vi "SerialCommand.vi"(4 "Received":refnum<k21>, 5 "ReceivedBuffer":refnum<k21>, 6 "Transmitted":refnum<k21>, 7 "Out":refnum<k21>, 8 "error in (no error)":errorcluster, 9 "CommandFIFO":refnum<k21>, 10 "Command":u8, 11 "Port":refnum<k21>) -> (0 "error out":errorcluster)   [LabVIEW 2023]
uses:
  <vilib>/rvi/DataTransferAndStorage/Container/Common/niFpgaContainerExecOnDevCompGetState.vi
  <vilib>/rvi/Emulation/niFpgaEmulationIsFPGAContextNoSignature.vi
  <vilib>/rvi/Emulation/niFpgaSctlEmulationGetInTimedLoop.vi
  <vilib>/rvi/errors/niFpgaSetErrorForExecOnDevCompSimple.vi
  <vilib>/rvi/eio/common/nirviEmuReportErrorAndStop.vi
  <vilib>/rvi/DataTransferAndStorage/Container/Common/niFpgaContainerGetUniqueNameForEmu.vi
  <vilib>/rvi/FIFO/Fifo_Resource/nirvififoEmulationSetSize.vi
  <vilib>/rvi/FIFO/Fifo_Resource/nirviFifoEmulationQueueMgr.vi
  <instcachedir>/0/nirviFifoEmulationQueueMgr_E5CAEC123FF24DC58D834DCA3CDAA9B5.lvgen/nirviFifoEmulationQueueMgr_E5CAEC123FF24DC58D834DCA3CDAA9B5_002.vi
  <vilib>/rvi/FIFO/Fifo_Resource/nirvififoEmulationDetermineInputValidOut.vi
  <vilib>/rvi/FIFO/Fifo_Resource/nirvififoEmulationCreateLock.vi
  <vilib>/rvi/Emulation/niFpgaProcessEmulError.vi
  <vilib>/rvi/FIFO/Fifo_Resource/nirvififoEmulationObtainLock.vi
  <vilib>/rvi/FIFO/Fifo_Resource/nirvififoEmulationReleaseLock.vi
  <vilib>/rvi/occurrence/nirviWaitOnOccurrenceBase.vi
  <vilib>/rvi/errors/nirviReportUnexpectedCaseInternalError.vi
  <vilib>/rvi/errors/nirviReportUnexpectedCaseInternalError (U32).vi
  <vilib>/Utility/error.llb/Clear Errors.vi
  <vilib>/eio/utilities/niEioResolveVilibRelativePath.vi
  <vilib>/rvi/interface/RandomDataEmulation/niFpgaRandomDataHandleErrors.vi
  <vilib>/rvi/Memory/Memory_Emulation/niFpgaMemoryEmulationCacheClearOnFirstRun.vi
  <vilib>/rvi/Memory/Memory_Emulation/nirvimemoryEmulationManagerCache_MakeExclusive.vi
  <vilib>/rvi/Memory/Memory_Emulation/niFpgaMemoryEmulationValidateCache.vi
  <vilib>/rvi/Memory/Memory_Emulation/nirvimemoryEmulationManagerCache_InsertValue.vi
  <vilib>/rvi/Memory/Memory_Emulation/nirvimemoryEmulationManagerCache_ReleaseExclusive.vi
  <vilib>/rvi/Memory/Memory_Emulation/nirvimemoryEmulationManagerCache_GetValue.vi
  <vilib>/rvi/Memory/Memory_Emulation/nirvimemoryEmulationManagerCache_SetValue.vi
  <vilib>/rvi/eio/common/nirviEmuTemplateMethod_errors.vi
  <vilib>/rvi/DataTransferAndStorage/Container/XNode/niFpgaContainer.xnode
  <vilib>/rvi/FIFO/Fifo_Resource/niFpgaFifoEmulationRefIn.vi
  <vilib>/rvi/DataTransferAndStorage/Register/Emulation/niFpgaRegisterEmulationRefIn.vi
  <vilib>/eio/EIOMethodNode/EIOMethodNode.xnode
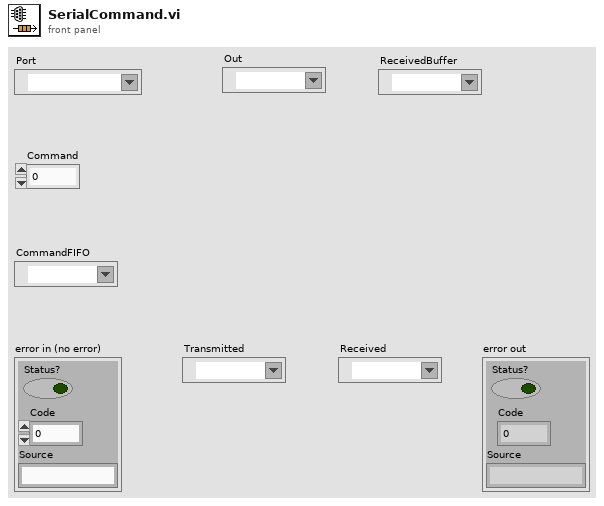
[diagram p1: front panel]
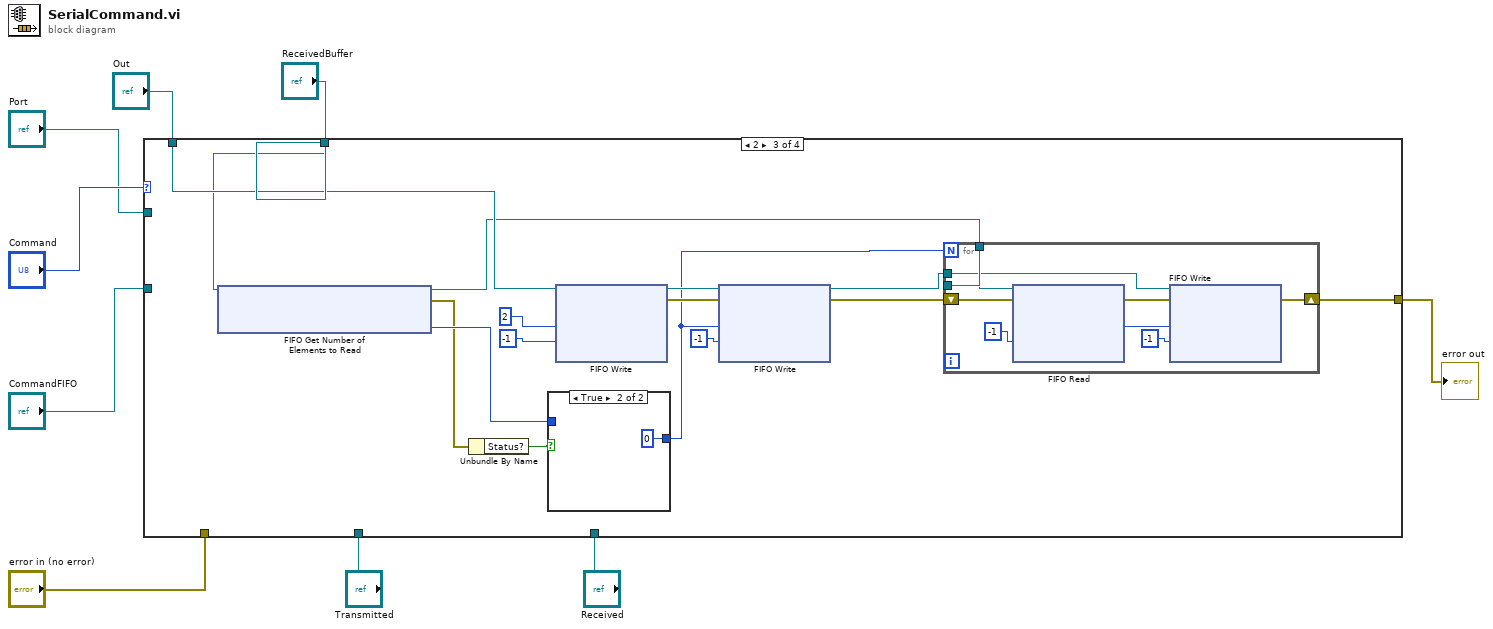
[diagram p0: block diagram]
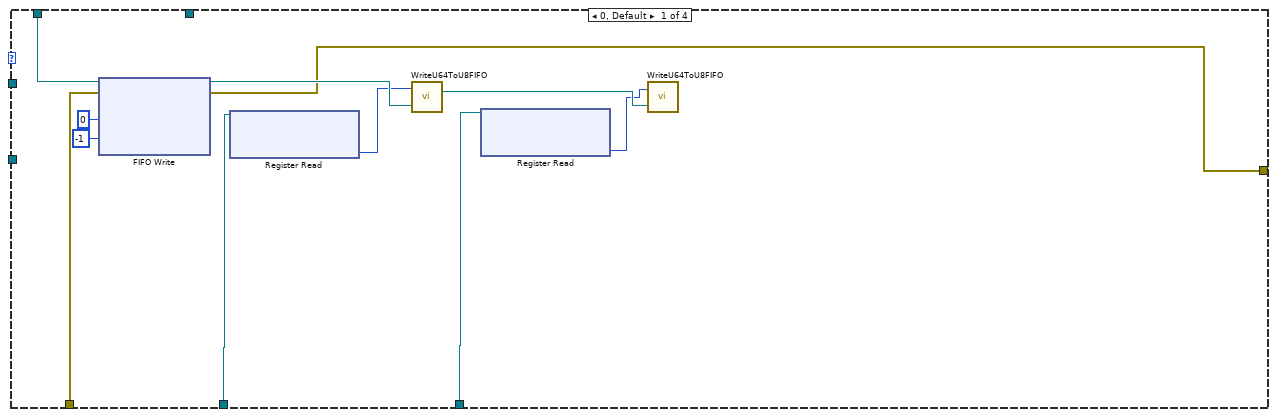
[diagram p2: hidden frame]
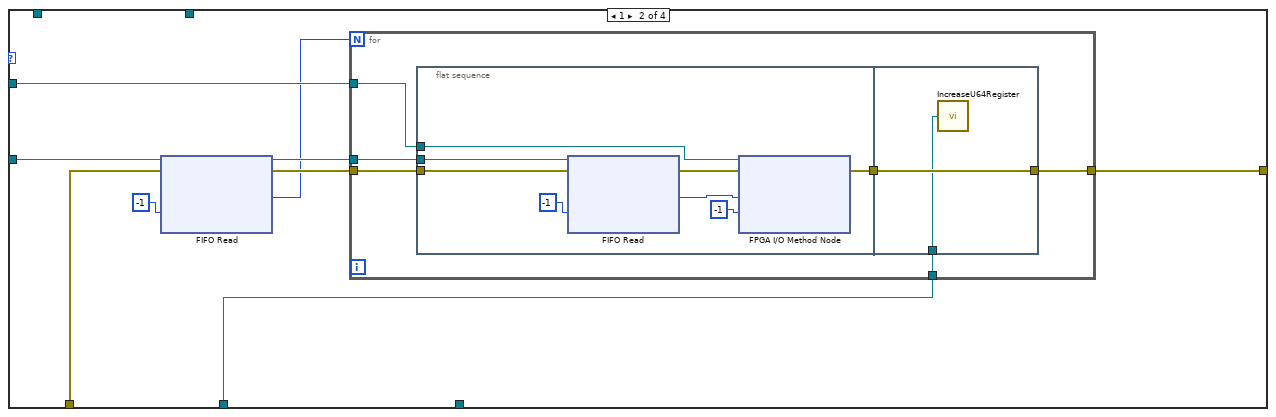
[diagram p3: hidden frame]
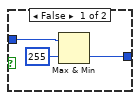
[diagram p4: hidden frame]
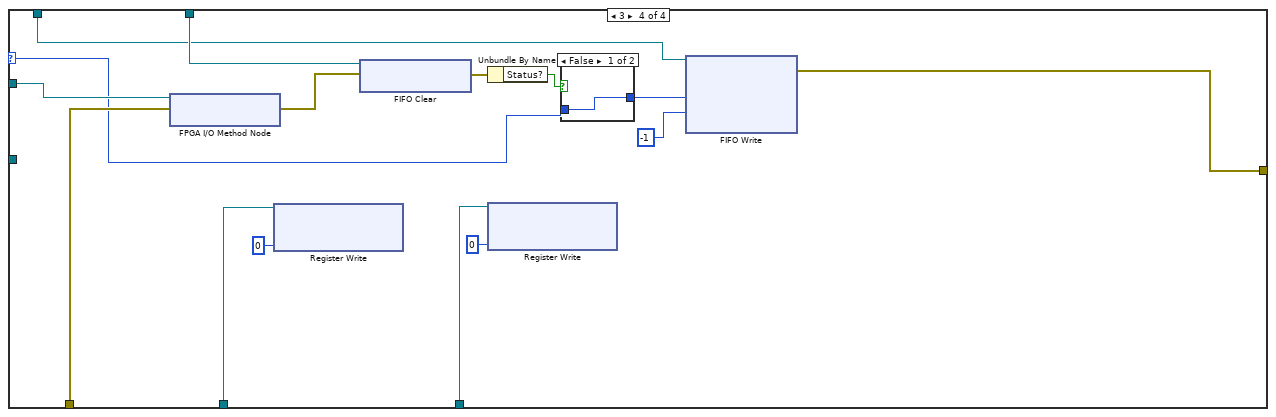
[diagram p5: hidden frame]
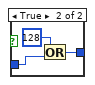
[diagram p6: hidden frame]
diagram:
  n1 = case shown="2" "Command" {
    selector: "Command" -> [_ _ _ w77]
    tunnel: "Port" -> [_ w29 _ w86]
    tunnel: [w10 w28 w60 w75] -> w7
    tunnel: "CommandFIFO" -> [_ w27 _ _]
    tunnel: "Received" -> [w16 _ _ w81]
    tunnel: "Transmitted" -> [w14 w21 _ w83]
    tunnel: "Out" -> [w12 _ w52 w85]
    tunnel: "ReceivedBuffer" -> [_ _ w51 w87]
    tunnel: "error in (no error)" -> [w11 w22 _ w79]
    frame 0, Default {
      n2 = xnode ("FIFO Write")("Element"=u8 0, "Timeout"=-1, "error in (no error)"=w11, "FIFO In"=w12) -> ("error out"=w10:errorcluster, "FIFO Out"=w20:refnum<k21>)  [unwired: 1 out]
      n3 = xnode ("Register Read")("Register In"=w14) -> ("Data"=w13:u64)  [unwired: 1 out]
      n4 = call "WriteU64ToU8FIFO.vi"("FIFO"=w20, "Value"=w13) -> ("FIFO"=w17:refnum<k21>)
      n5 = xnode ("Register Read")("Register In"=w16) -> ("Data"=w15:u64)  [unwired: 1 out]
      n6 = call "WriteU64ToU8FIFO.vi"("FIFO"=w17, "Value"=w15) -> ()  [unwired: 1 out]
    }
    frame 1 {
      n7 = xnode ("FIFO Read")("Timeout"=-1, "error in (no error)"=w22, "FIFO In"=w27) -> ("Element"=w23:u8, "error out"=w25:errorcluster, "FIFO Out"=w26:refnum<k21>)  [unwired: 1 out]
      n8 = for {
        N: w23 -> [_]
        tunnel: w26 -> [w34]
        tunnel: w29 -> [w35]
        tunnel: [w33] -> w28
        tunnel: w25 -> [w31]
        tunnel: w21 -> [w30]
        n9 = flat-sequence {
          tunnel: w35 -> [w41]
          tunnel: w31 -> [w38]
          tunnel: w34 -> [w37]
          tunnel: [w36] -> w32
          tunnel: [w45] -> w33
          tunnel: w32 -> [w45]
          tunnel: w30 -> [w44]
          frame #0 {
            n10 = xnode ("FIFO Read")("Timeout"=-1, "error in (no error)"=w38, "FIFO In"=w37) -> ("Element"=w42:u8, "error out"=w43:errorcluster)  [unwired: 2 out]
            n11 = xnode "FPGA I/O Method Node"("error in"=w43, "FPGA I/O In"=w41, "Data"=w42, "Timeout (ms)"=-1) -> ("error out"=w36:errorcluster)  [unwired: 2 out]
          }
          frame #1 {
            n12 = call "IncreaseU64Register.vi"("Register In"=w44) -> ()  [unwired: 1 out]
          }
        }
      }
    }
    frame 2 {
      n13 = xnode ("FIFO Get Number of Elements to Read")("FIFO In"=w51) -> ("Number of Elements to Read"=w50:u32, "error out"=w47:errorcluster, "FIFO Out"=w48:refnum<k21>)  [unwired: 1 in]
      n14 = Unbundle By Name(w47) -> ("Status?"=w46:bool)
      n15 = case shown="True" w46 {
        tunnel: w50 -> [w63 _]
        tunnel: [w62 u32 0] -> w49
        frame False {
          n16 = Max & Min(x=w63, y=u32 255) -> (min(x,y)=w62:u32)  [unwired: 1 out]
        }
        frame True {
        }
      }
      n17 = xnode ("FIFO Write")("Element"=u8 2, "Timeout"=-1, "FIFO In"=w52) -> ("error out"=w54:errorcluster, "FIFO Out"=w57:refnum<k21>)  [unwired: 1 in, 1 out]
      n18 = xnode ("FIFO Write")("Element"=w49, "Timeout"=-1, "error in (no error)"=w54, "FIFO In"=w57) -> ("error out"=w53:errorcluster, "FIFO Out"=w56:refnum<k21>)  [unwired: 1 out]
      n19 = for {
        N: w49 -> [_]
        tunnel: w56 -> [w72]
        tunnel: w48 -> [_]
        shift-right: [w68] -> w60
        shift-left: w53 -> [w70]
        tunnel: w48 -> [w65]
        n20 = xnode ("FIFO Read")("Timeout"=-1, "error in (no error)"=w70, "FIFO In"=w65) -> ("Element"=w67:u8, "error out"=w69:errorcluster)  [unwired: 2 out]
        n21 = xnode ("FIFO Write")("Element"=w67, "Timeout"=-1, "error in (no error)"=w69, "FIFO In"=w72) -> ("error out"=w68:errorcluster)  [unwired: 2 out]
      }
    }
    frame 3 {
      n22 = xnode "FPGA I/O Method Node"("error in"=w79, "FPGA I/O In"=w86) -> ("error out"=w78:errorcluster)  [unwired: 1 out]
      n23 = xnode ("Register Write")("Data"=u64 0, "Register In"=w83) -> ()  [unwired: 1 out]
      n24 = xnode ("FIFO Clear")("error in (no error)"=w78, "FIFO In"=w87) -> ("error out"=w74:errorcluster)  [unwired: 1 out]
      n25 = Unbundle By Name(w74) -> ("Status?"=w73:bool)
      n26 = xnode ("Register Write")("Data"=u64 0, "Register In"=w81) -> ()  [unwired: 1 out]
      n27 = case shown="False" w73 {
        tunnel: w77 -> [w88 w91]
        tunnel: [w88 w89] -> w76
        frame False {
        }
        frame True {
          n28 = Or(x=i16 128, y=w91) -> (x .or. y?=w89:i16)
        }
      }
      n29 = xnode ("FIFO Write")("Element"=w76, "Timeout"=-1, "FIFO In"=w85) -> ("error out"=w75:errorcluster)  [unwired: 1 in, 2 out]
    }
  }
  "error out" <- w7
